vi "instrumentProperties_channel_attenuatorState.vi"(6 "poll write":bool, 8 "error in (no error)":errorcluster, 9 "readWrite":enum16{"read", "write"}(ring), 10 "attenFilter_active":bool, 11 "OSAchannel in":refnum<class "OSAchannel.lvclass">) -> (0 "error out":errorcluster, 1 "FTSLib status":i32, 2 "attenFilter_active read":bool, 3 "OSAchannel out":refnum<class "OSAchannel.lvclass">, 4 "poll timeOut":bool)   [LabVIEW 2010, in "OSAchannel.lvclass"]
uses:
  OSAchannel.lvclass
  OSAchannel.lvclass/OSAchannel.ctl
  FTSLib.dll
  OSA20X_misc.lvlib
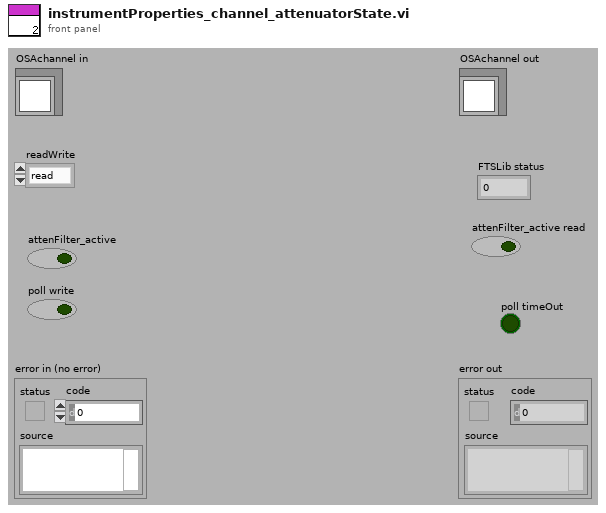
[diagram p1: front panel]
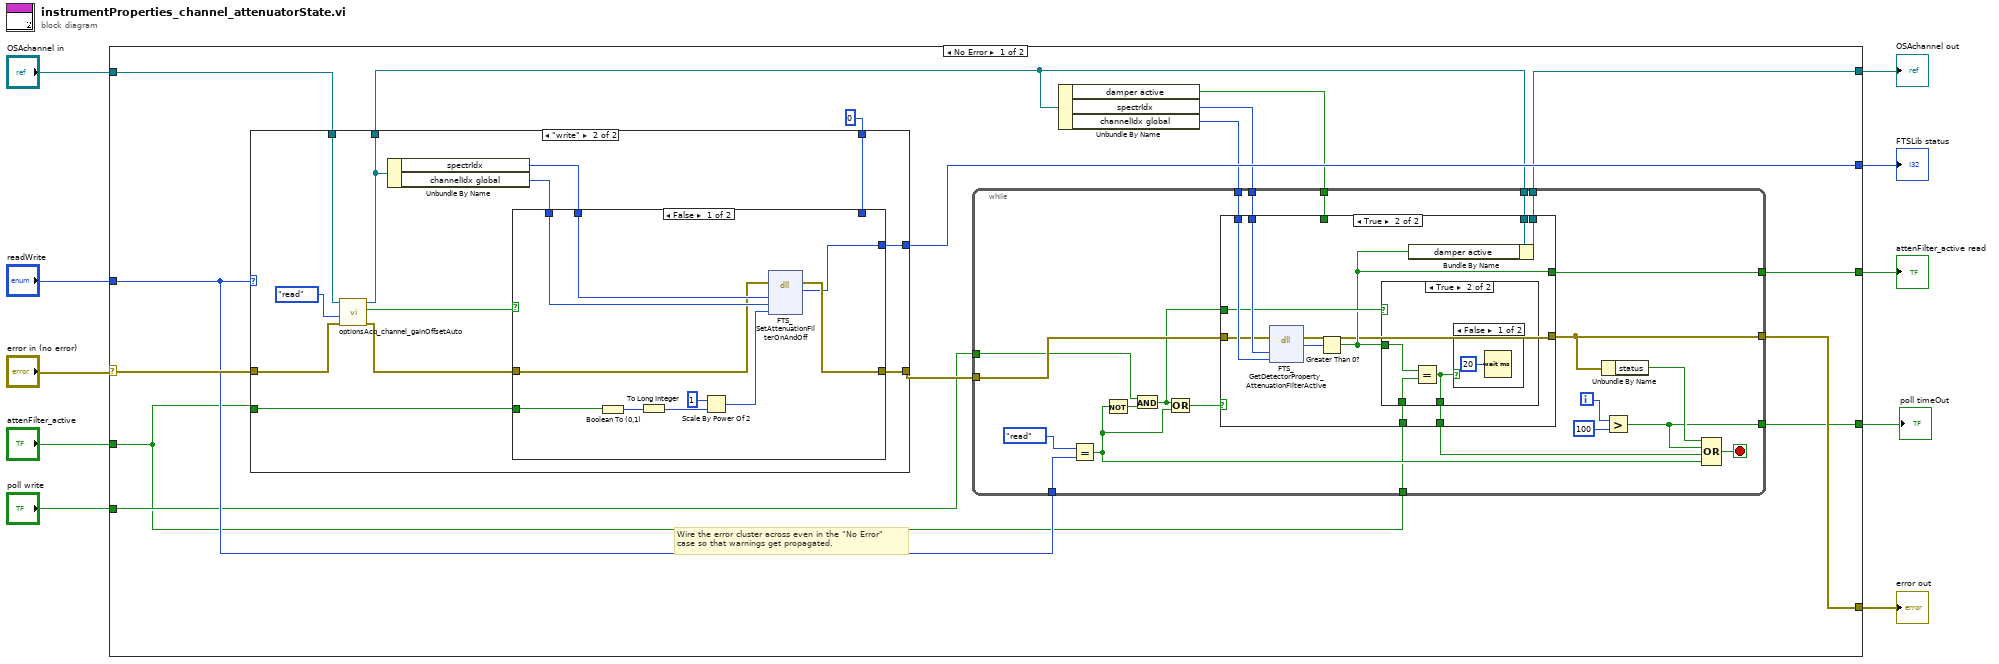
[diagram p0: block diagram]
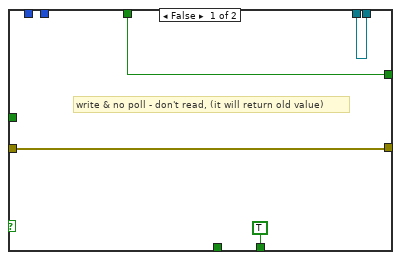
[diagram p2: hidden frame]
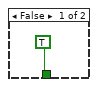
[diagram p3: hidden frame]
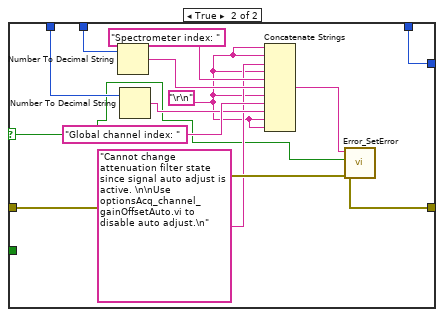
[diagram p6: hidden frame]
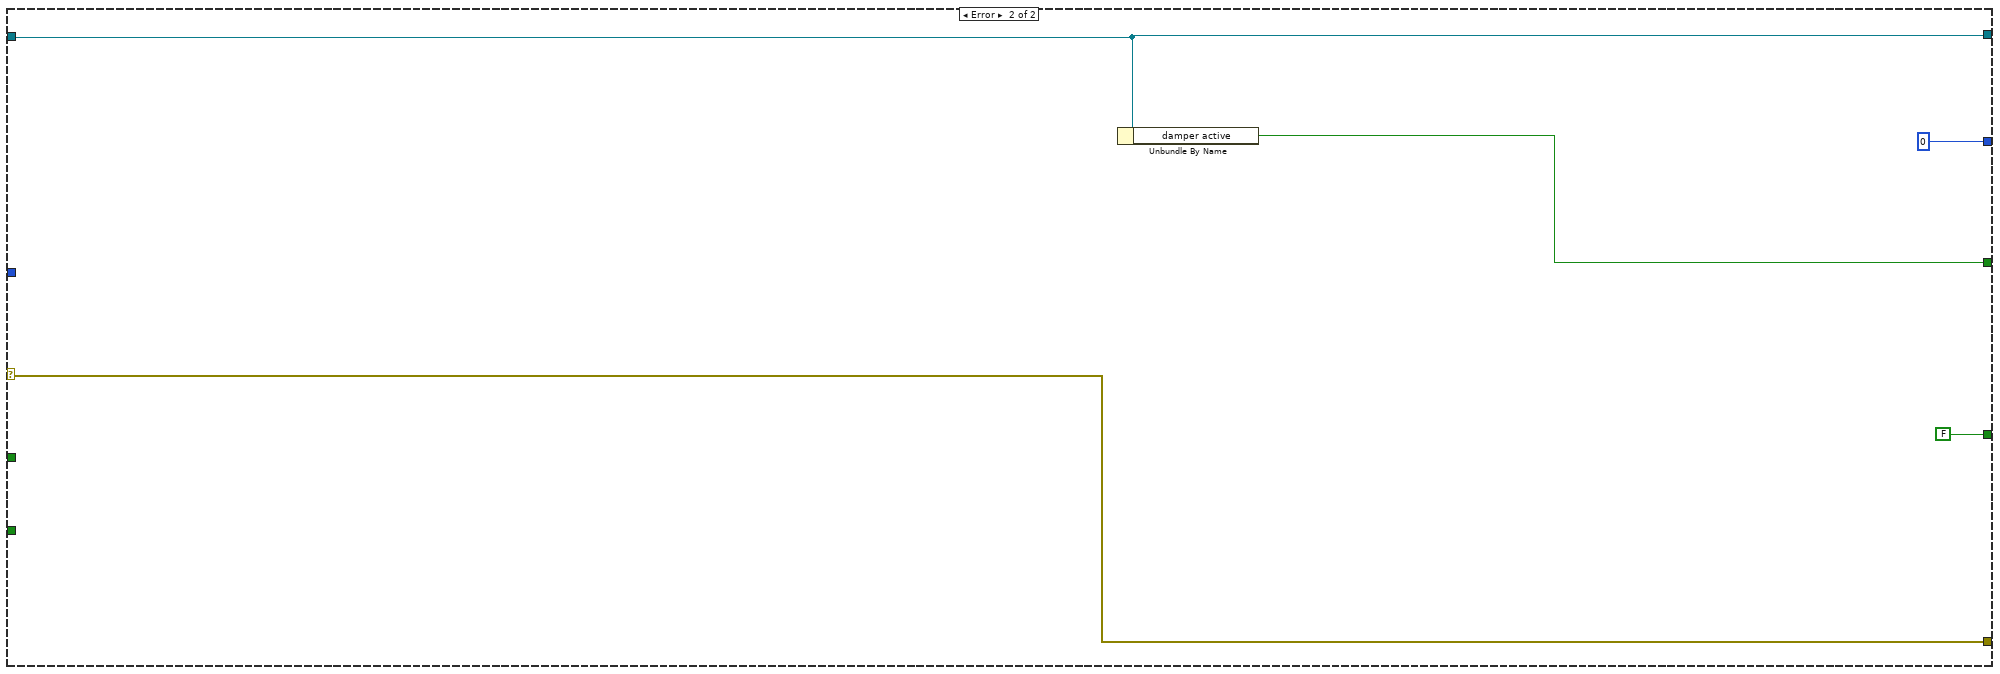
[diagram p7: hidden frame]
diagram:
  n1 = case shown="No Error" "error in (no error)" {
    selector: "error in (no error)" -> [w26 w111]
    tunnel: [w14 w111] -> w9
    tunnel: [w16 w110] -> w7
    tunnel: "OSAchannel in" -> [w12 w110]
    tunnel: "readWrite" -> [w23 _]
    tunnel: "attenFilter_active" -> [w18 _]
    tunnel: [w25 0 ("result")] -> w4
    tunnel: "poll write" -> [w19 _]
    tunnel: [w17 w109] -> w2
    tunnel: [w13 FALSE] -> w1
    frame No Error {
      # "Wire the error cluster across even in the \"No Error\"\ncase so that warnings get propagated."
      n2 = case shown="\"write\"" w23 {
        tunnel: [w71 w82] -> w25
        tunnel: w26 -> [w70 w80]
        tunnel: [w70 w83] -> w20
        tunnel: w18 -> [_ w81]
        tunnel: 0 ("result") -> [w71 w76]
        tunnel: w12 -> [w69 w75]
        tunnel: [w69 w74] -> w11
        frame Default {
        }
        frame "write" {
          n3 = call "optionsAcq_channel_gainOffsetAuto.vi"("error in (no error)"=w80, "readWrite"=enum16{"read", "write"}."read", "OSAchannel in"=w75) -> ("error out"=w78:errorcluster, "auto read"=w77:bool, "OSAchannel out"=w74:refnum<class "OSAchannel.lvclass">)  [unwired: 5 in, 1 out]
          n4 = Unbundle By Name(w74) -> ("spectrIdx"=w72:u16, "channelIdx global"=w73:u16)
          n5 = case shown="False" w77 {
            selector: w77 -> [_ w94]
            tunnel: w73 -> [w93 w103]
            tunnel: w72 -> [w92 w104]
            tunnel: w78 -> [w91 w106]
            tunnel: [w90 w105] -> w83
            tunnel: [w89 w95] -> w82
            tunnel: w81 -> [w84 _]
            tunnel: w76 -> [_ w95]
            frame False {
              n6 = Boolean To (0,1)(Boolean=w84) -> (0, 1=w86:i16)
              n7 = To Long Integer(number=w86) -> (32bit integer=w87:i32)
              n8 = Scale By Power Of 2(n=1, x=w87) -> (x*2^n=w85:i32)
              n9 = dll-call lib="FTSLib.dll" fn="FTS_SetAttenuationFilterOnAndOff"(error in=w91, "spectrIdx"=w92, "channeldx"=w93, "filterStatus"=w85) -> (error out=w90:errorcluster, "result"=w89:i32)  [unwired: 5 in, 1 out]
            }
            frame True {
              w96 = "\r\n"
              n10 = Number To Decimal String(number=w104) -> (decimal integer string=w101:string)  [unwired: 1 in]
              n11 = Number To Decimal String(number=w103) -> (decimal integer string=w99:string)  [unwired: 1 in]
              n12 = Concatenate Strings(w96, w96, "Cannot change attenuation filter state since signal auto adjust is active. \n\nUse optionsAcq_channel_gainOffsetAuto.vi to disable auto adjust.\n" ("source(\"\")"), w96, "Spectrometer index: " ("string"), w101, w96, "Global channel index: " ("string"), w99, w96, w96) -> (w97:string)
              n13 = call "Error_SetError.vi"("error in"=w106, "status (true)"=w94, "source(\"\")"=w97) -> ("error out"=w105:errorcluster)  [unwired: 4 in]
            }
          }
        }
      }
      n14 = Unbundle By Name(w11) -> ("damper active"=w15:bool, "spectrIdx"=w21:u16, "channelIdx global"=w22:u16)
      n15 = while {
        tunnel: w23 -> [w48]
        tunnel: w22 -> [w45]
        tunnel: w21 -> [w44]
        tunnel: w20 -> [w43]
        tunnel: w19 -> [w39]
        tunnel: w18 -> [w38]
        tunnel: [w35] -> w17
        tunnel: w11 -> [w34]
        tunnel: [w33] -> w16
        tunnel: w15 -> [w32]
        tunnel: [w28] -> w14
        tunnel: [w27] -> w13
        i -> [w31]
        stop <- w46 stop-if-true
        n16 = Equal?(x=enum16{"read", "write"}."read", y=w48) -> (x = y?=w42:bool)
        n17 = Not(x=w42) -> (.not. x?=w41:bool)
        n18 = And(x=w39, y=w41) -> (x .and. y?=w37:bool)
        n19 = Or(x=w37, y=w42) -> (x .or. y?=w40:bool)
        n20 = case shown="True" w40 {
          tunnel: w45 -> [_ w62]
          tunnel: w44 -> [_ w61]
          tunnel: w43 -> [w49 w60]
          tunnel: w38 -> [_ w59]
          tunnel: w37 -> [_ w58]
          tunnel: [TRUE w57] -> w36
          tunnel: [w50 w54] -> w35
          tunnel: w34 -> [w51 w56]
          tunnel: [w51 w55] -> w33
          tunnel: w32 -> [w50 _]
          tunnel: [w49 w53] -> w28
          frame False {
            # "write & no poll - don't read, (it will return old value)"
          }
          frame True {
            n21 = dll-call lib="FTSLib.dll" fn="FTS_GetDetectorProperty_AttenuationFilterActive"(error in=w60, "spectrIdx"=w61, "channeldx"=w62) -> (error out=w53:errorcluster, "attenuatorActive"=w63:i32)  [unwired: 4 in, 1 out]
            n22 = Greater Than 0?(x=w63) -> (x > 0?=w54:bool)
            n23 = case shown="True" w58 {
              tunnel: w54 -> [_ w66]
              tunnel: w59 -> [_ w67]
              tunnel: [TRUE w65] -> w57
              frame False {
              }
              frame True {
                n24 = Equal?(x=w66, y=w67) -> (x = y?=w65:bool)
                n25 = case shown="False" w65 {
                  frame False {
                    n26 = Wait (ms)(milliseconds to wait=u32 20) -> ()  [unwired: 1 out]
                  }
                  frame True {
                  }
                }
              }
            }
            n27 = Bundle By Name(cluster=w56, "damper active"=w54) -> (w55:refnum<class "OSAchannel.lvclass">)
          }
        }
        n28 = Unbundle By Name(w28) -> ("status"=w29:bool)
        n29 = Greater?(x=w31, y=100) -> (0:w27:bool)
        n30 = Compound Arithmetic op=OR(w29, w27, w36, w42) -> (w46:bool)
      }
    }
    frame Error {
      n31 = Unbundle By Name(w110) -> ("damper active"=w109:bool)
    }
  }
  "error out" <- w9
  "OSAchannel out" <- w7
  "attenFilter_active read" <- w2
  "FTSLib status" <- w4
  "poll timeOut" <- w1
